vi "Module.Initializer.vi"(4 "StatusTxtBx":refnum<vi>, 5 "Menu Ref":refnum<k9>, 6 "Pane":refnum<vi>, 7 "Main Tab":refnum<vi>, 8 "error in":errorcluster, 9 "Self Ref":refnum<vi>, 10 "Module Config":T3, 11 "SW Rev":T2) -> (0 "error out":errorcluster, 3 "Sys":T1)   [LabVIEW 2024, in "EQMF.lvlib" / "Module Utils.lvlib"]
uses:
  Module Utils.lvlib
  Module Config.ctl
  Queues/Q.Element.ctl
  Module.Working Dirs.ctl
  Module.SW Version Info.ctl
  Module Sys Info.ctl
  Config/Stored Controls/Class.SaveCtrls.lvclass
  Event Log/Event Notification/Event Notification.lvclass
  Config/App Data/Class.AppData.lvclass
  Subscription/Subscription.lvclass
  Queues/Queue Utils.lvlib
  Controls/Controls.lvlib
  Event Log/Event Log.lvlib
  Scheduler/Scheduler.lvlib
  Menu/Menu Utils.lvlib
  Config/Config Utils.lvlib
panel:
  # "Name, PN, Version, Note"
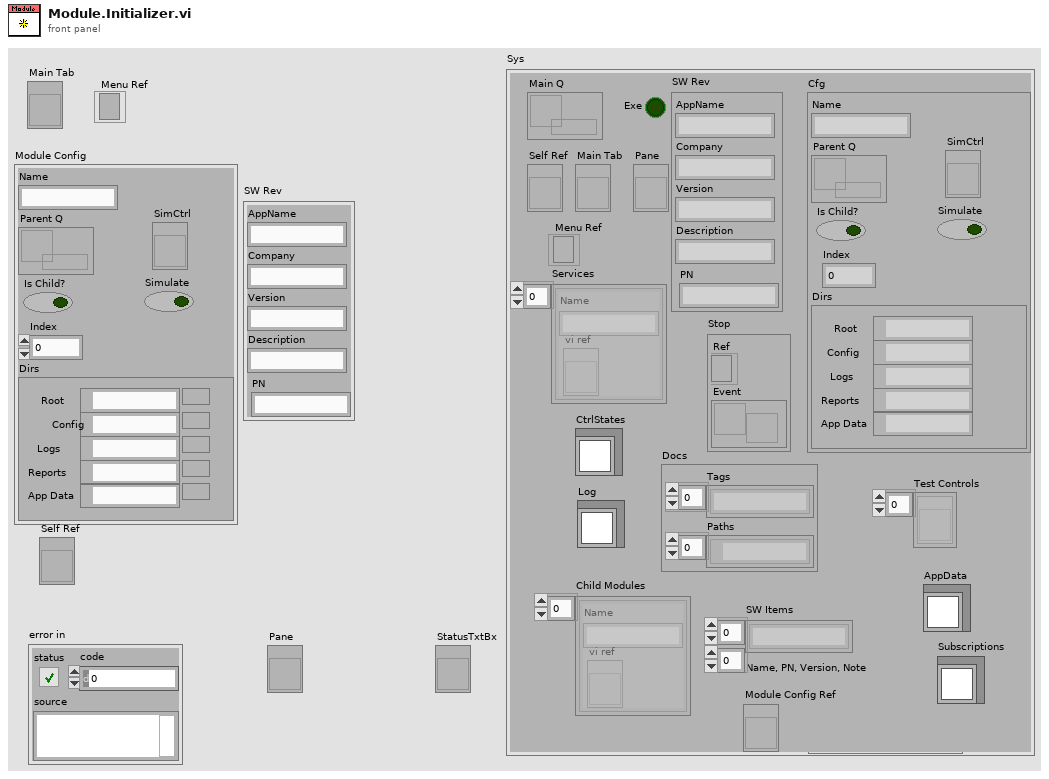
[diagram p1: front panel]
types:
  T1 = typedef "EQMF.lvlib/Module Utils.lvlib/Module Sys Info.ctl" = cluster{"Main Q":refnum<queue>, "Exe":bool, "SW Rev":T2, "Self Ref":refnum<vi>, "Main Tab":refnum<vi>, "Pane":refnum<vi>, "Stop":cluster{"Ref":refnum<event-registration>, "Event":refnum<user-event>}, "Cfg":T3, "Services":cluster{"Name":string, "vi ref":refnum<vi>}[], "Menu Ref":refnum<k9>, "CtrlStates":refnum<class "Class.SaveCtrls.lvclass">, "Docs":cluster{"Tags":string[], "Paths":path[]}, "Log":refnum<class "Event Notification.lvclass">, "Test Controls":refnum<vi>[], "Child Modules":cluster{"Name":string, "vi ref":refnum<vi>}[], "SW Items":string[][], "AppData":refnum<class "Class.AppData.lvclass">, "Subscriptions":refnum<class "Subscription.lvclass">, "Module Config Ref":refnum<vi>}
  T2 = typedef "EQMF.lvlib/Module Utils.lvlib/Module.SW Version Info.ctl" = cluster{"AppName":string, "Company":string, "Version":string, "Description":string, "PN":string}
  T3 = typedef "EQMF.lvlib/Module Utils.lvlib/Module Config.ctl" = cluster{"Name":string, "Parent Q":refnum<queue>, "Is Child?":bool, "Index":i32, "Dirs":T4, "Simulate":bool, "SimCtrl":refnum<vi>}
  T4 = typedef "EQMF.lvlib/Module Utils.lvlib/Module.Working Dirs.ctl" = cluster{"Root":path, "Config":path, "Logs":path, "Reports":path, "App Data":path}
  T5 = enum32{"invalid app kind", "Development System", "Run Time System", "Student Edition", "Embedded LabVIEW", "Evaluation", "Custom"}
  T6 = typedef "LVMenuShortCut.ctl" = cluster{"include Shift key?":bool, "include Ctrl key?":bool, "shortcut key":string}
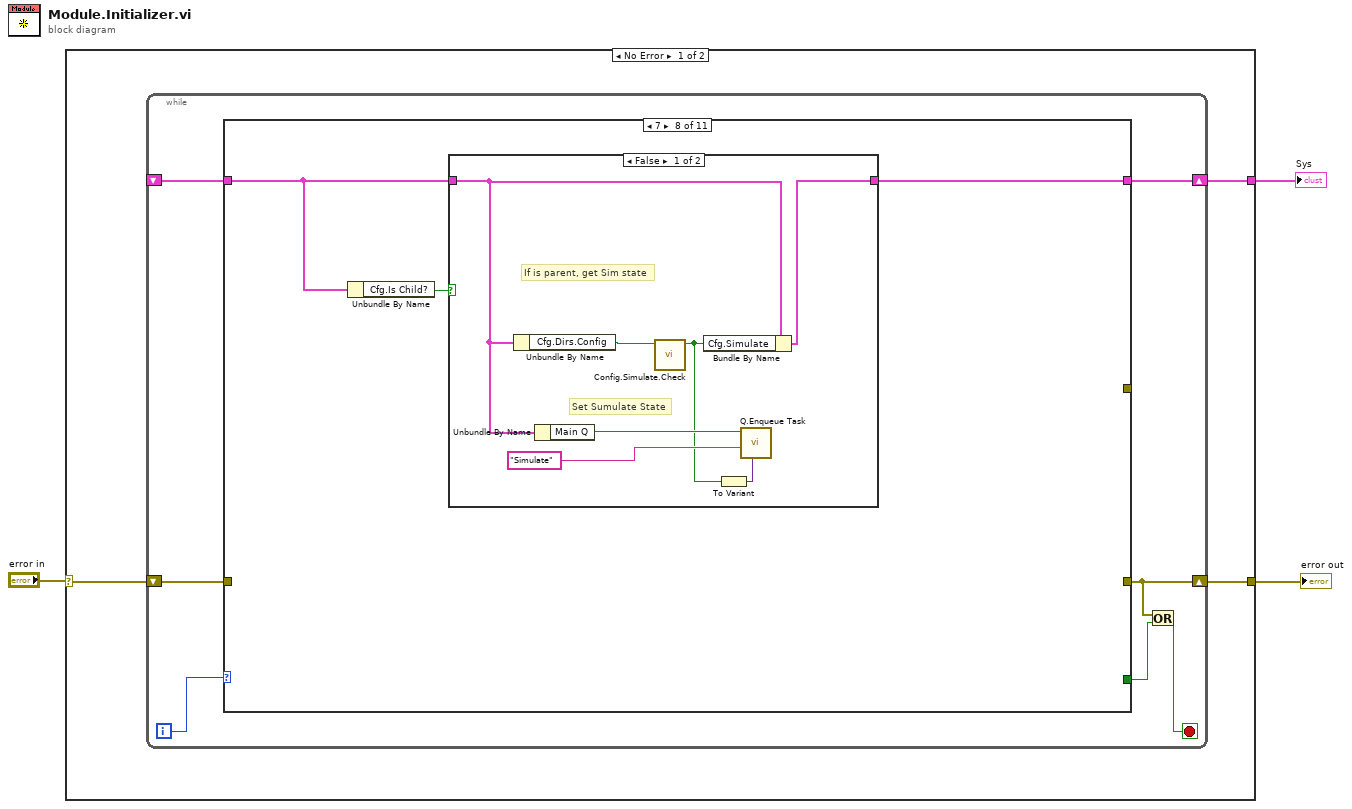
[diagram p0: block diagram]
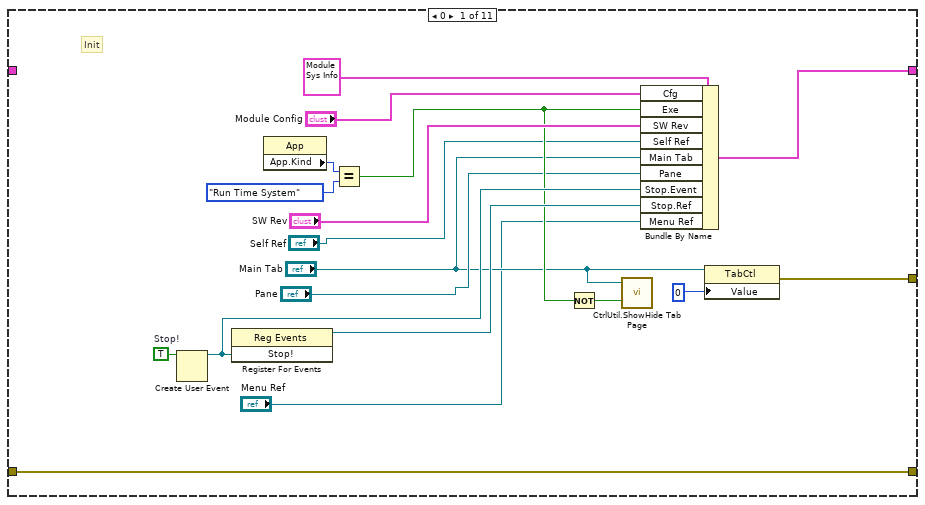
[diagram p2: hidden frame]
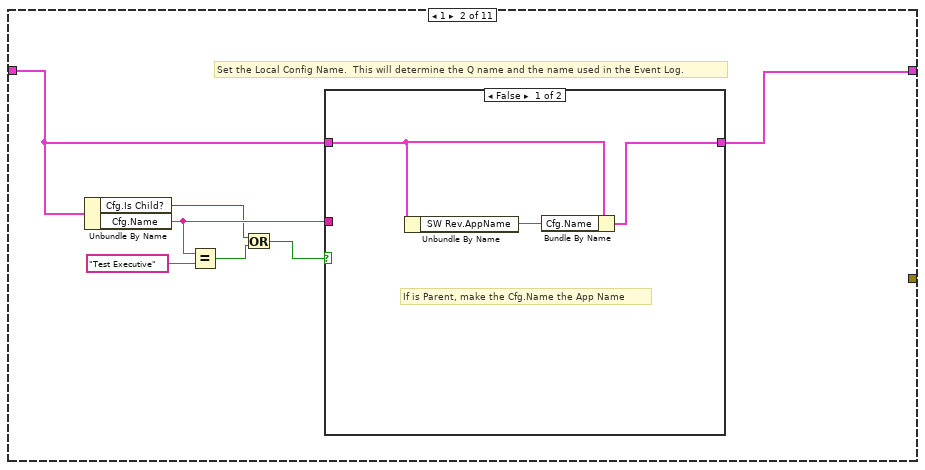
[diagram p3: hidden frame]
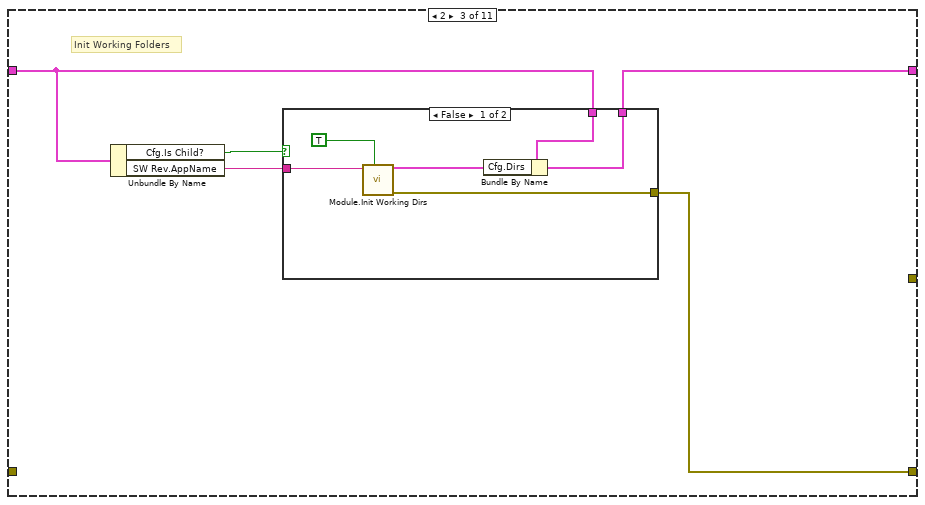
[diagram p5: hidden frame]
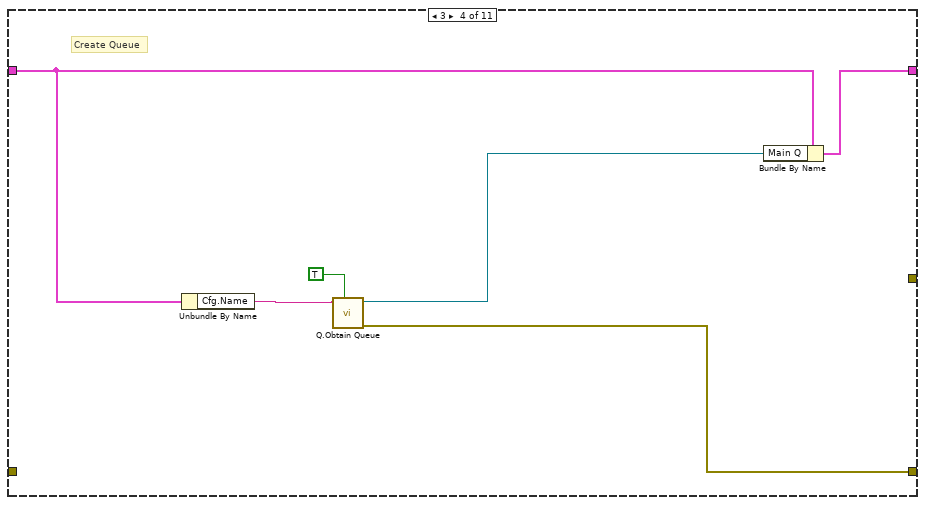
[diagram p7: hidden frame]
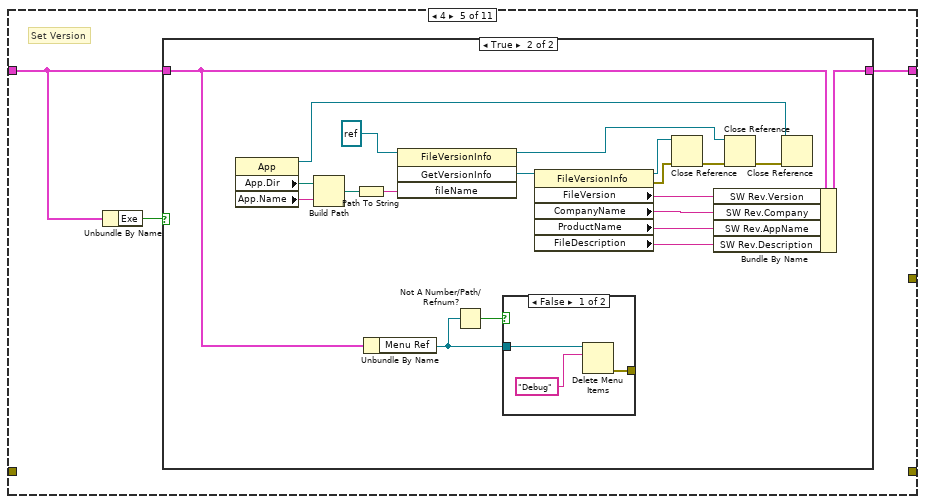
[diagram p8: hidden frame]
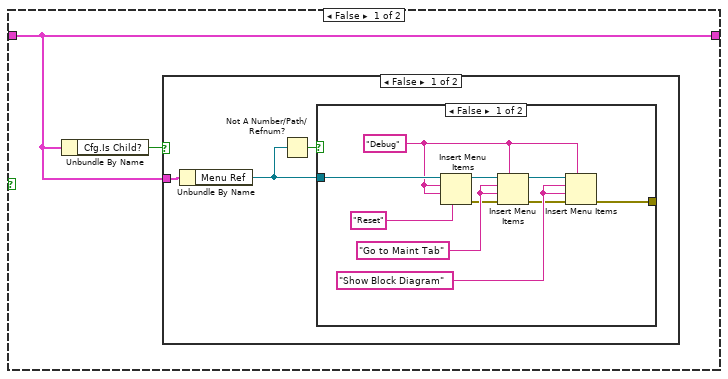
[diagram p9: hidden frame]
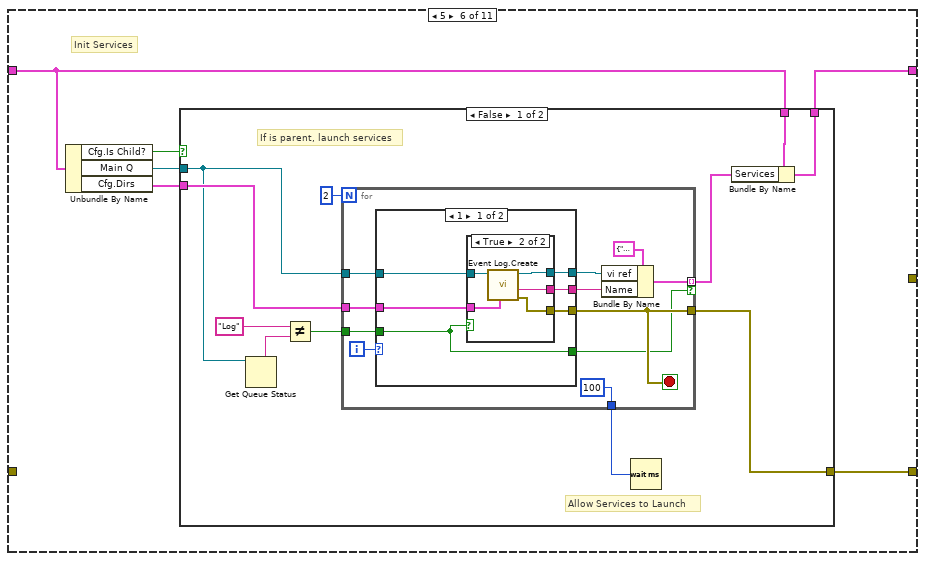
[diagram p13: hidden frame]
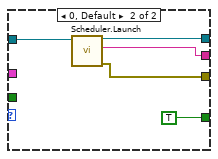
[diagram p15: hidden frame]
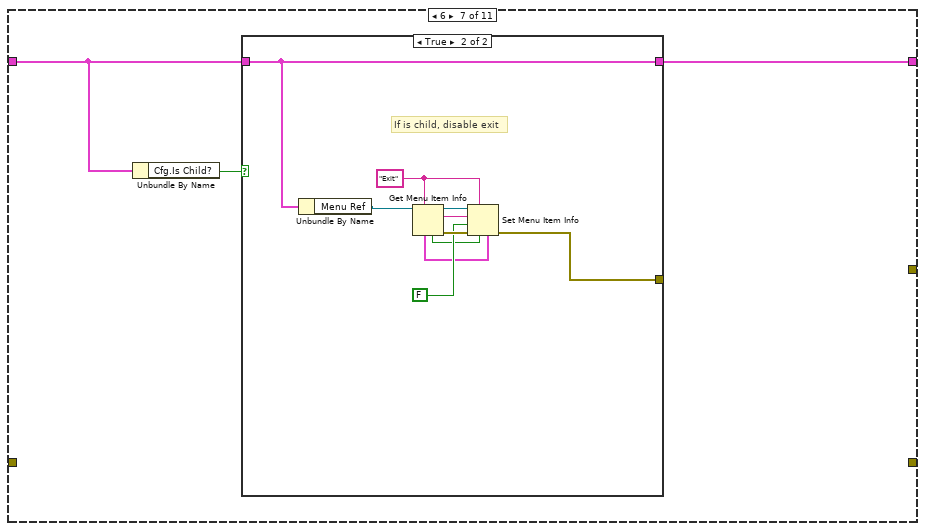
[diagram p17: hidden frame]
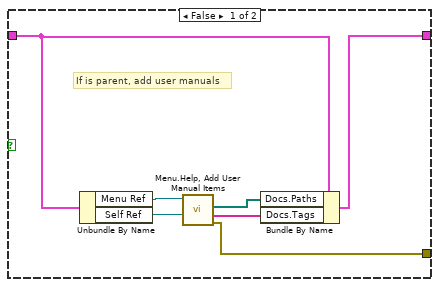
[diagram p18: hidden frame]
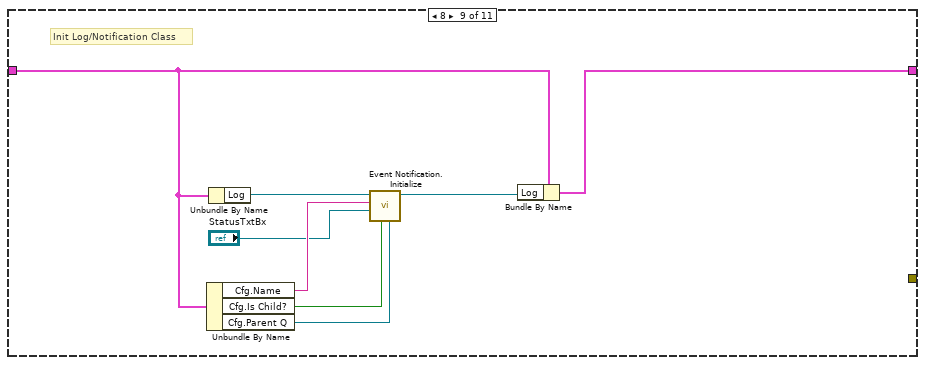
[diagram p20: hidden frame]
diagram:
  n1 = case shown="No Error" "error in" {
    selector: "error in" -> [w6 w197]
    tunnel: [w4 w197] -> w3
    tunnel: [w5 _] -> w1
    frame No Error {
      n2 = while {
        shift-right: [w7] -> w5
        shift-left: _ -> [w12]
        shift-right: [w8] -> w4
        shift-left: w6 -> [w9]
        i -> [w13]
        stop <- w10 stop-if-true
        n3 = case shown="7" w13 {
          tunnel: w12 -> [_ w36 w45 w56 w62 w106 w148 w168 w184 w193 w194]
          tunnel: [_ _ _ _ _ _ _ _ _ _ TRUE] -> w11
          tunnel: w9 -> [w22 _ _ _ _ _ _ _ _ _ w195]
          tunnel: [w22 _ w43 w58 _ w104 _ _ _ _ w195] -> w8
          tunnel: [w26 w35 w44 w60 w61 w105 w149 w169 w185 w192 w194] -> w7
          tunnel: [w15 _ _ _ _ _ _ _ _ _ _] -> _
          frame 0 {
            w25 = TRUE  # Stop!
            # "Init"
            n4 = Create User Event(user event datatype=w25) -> (user event=w24:refnum<user-event>)  [unwired: 1 in, 1 out]
            n5 = register-events(w24) -> (reference out=w23:refnum<event-registration>)  [unwired: 2 in, 1 out]
            n6 = property class="App"() -> ("App.Kind"=w28:T5)  [unwired: 2 in, 2 out]
            n7 = Equal?(x=w28, y=T5."Run Time System" ("Application:Kind")) -> (x = y?=w20:bool)
            n8 = Not(x=w20) -> (.not. x?=w21:bool)
            n9 = call "CtrlUtil.ShowHide Tab Page.vi"("Show"=w21, "Tab Control"="Main Tab") -> ()  [unwired: 3 in]
            n10 = Bundle By Name(cluster=T1 {"Main Q"=refnum, "Exe"=FALSE, "SW Rev"={"AppName"="", "Company"="", "Version"="", "Description"="", "PN"=""}, "Self Ref"=refnum, "Main Tab"=refnum, "Pane"=refnum, "Stop"={"Ref"=refnum, "Event"=refnum}, "Cfg"={"Name"="", "Parent Q"=refnum, "Is Child?"=FALSE, "Index"=0, "Dirs"={"Root"=path "", "Config"=path "", "Logs"=path "", "Reports"=path "", "App Data"=path ""}, "Simulate"=FALSE, "SimCtrl"=refnum}, "Services"=[], "Menu Ref"=refnum, "CtrlStates"=refnum, "Docs"={"Tags"=[], "Paths"=[]}, "Log"=refnum, "Test Controls"=[], "Child Modules"=[], "SW Items"=[], "AppData"=refnum, "Subscriptions"=refnum, "Module Config Ref"=refnum} ("Sys"), "Cfg"="Module Config", "Exe"=w20, "SW Rev"="SW Rev", "Self Ref"="Self Ref", "Main Tab"="Main Tab", "Pane"="Pane", "Stop.Event"=w24, "Stop.Ref"=w23, "Menu Ref"="Menu Ref") -> (w26:T1)
            n11 = property class="TabCtl"(reference="Main Tab", "Value"=0) -> (error out=w15:errorcluster)  [unwired: 1 in, 1 out]
          }
          frame 1 {
            # "Set the Local Config Name.  This will determine the Q name and the name used in the Event Log."
            n12 = Unbundle By Name(w36) -> ("Cfg.Is Child?"=w33:bool, "Cfg.Name"=w37:string)
            n13 = Equal?(x=w37, y="Test Executive") -> (x = y?=w34:bool)
            n14 = Or(x=w33, y=w34) -> (x .or. y?=w32:bool)
            n15 = case shown="False" w32 {
              tunnel: w37 -> [_ _]
              tunnel: w36 -> [w41 w42]
              tunnel: [w39 w42] -> w35
              frame False {
                # "If is Parent, make the Cfg.Name the App Name"
                n16 = Unbundle By Name(w41) -> ("SW Rev.AppName"=w40:string)
                n17 = Bundle By Name(cluster=w41, "Cfg.Name"=w40) -> (w39:T1)
              }
              frame True {
                # "If is Child\n  Use Config name assigned\nIf is Test Executive:\n   No change to Cfg.Name"
              }
            }
          }
          frame 2 {
            # "Init Working Folders"
            n18 = Unbundle By Name(w45) -> ("Cfg.Is Child?"=w46:bool, "SW Rev.AppName"=w47:string)
            n19 = case shown="False" w46 {
              tunnel: w47 -> [w53 _]
              tunnel: [w52 _] -> w43
              tunnel: w45 -> [w50 w54]
              tunnel: [w49 w54] -> w44
              frame False {
                n20 = call "Module.Init Working Dirs.vi"("Public Docs"=TRUE, "App Name"=w53) -> ("error out"=w52:errorcluster, "Working Dirs"=w51:T4)  [unwired: 8 in]
                n21 = Bundle By Name(cluster=w50, "Cfg.Dirs"=w51) -> (w49:T1)
              }
              frame True {
              }
            }
          }
          frame 3 {
            # "Create Queue"
            n22 = Unbundle By Name(w56) -> ("Cfg.Name"=w55:string)
            n23 = call "Q.Obtain Queue.vi"("Enqueue Init"=TRUE, "Q Name"=w55) -> ("error out"=w58:errorcluster, "Q Out"=w59:refnum<queue>)  [unwired: 7 in, 1 out]
            n24 = Bundle By Name(cluster=w56, "Main Q"=w59) -> (w60:T1)
          }
          frame 4 {
            # "Set Version"
            n25 = Unbundle By Name(w62) -> ("Exe"=w63:bool)
            n26 = case shown="True" w63 {
              tunnel: w62 -> [w65 w82]
              tunnel: [w65 w97] -> w61
              frame False {
                n27 = Unbundle By Name(w65) -> ("Cfg.Is Child?"=w64:bool)
                n28 = case shown="False" w64 {
                  tunnel: w65 -> [w68 _]
                  frame False {
                    n29 = Unbundle By Name(w68) -> ("Menu Ref"=w66:refnum<k9>)
                    n30 = Not A Number/Path/Refnum?(number/path/refnum=w66) -> (NaN/Path/Refnum?=w67:bool)
                    n31 = case shown="False" w67 {
                      tunnel: w66 -> [w78 _]
                      tunnel: [w69 _] -> _
                      frame False {
                        w72 = "Show Block Diagram" ("menu tag")
                        w73 = "Go to Maint Tab" ("menu tag")
                        w74 = "Debug" ("menu tag")
                        n32 = Insert Menu Items(4:"Reset" ("after item"), 7:w74, 8:w74, 9:w78) -> (0:w71:errorcluster, 3:w76:refnum<k9>)  [unwired: 2 in, 1 out]
                        n33 = Insert Menu Items(5:w74, 6:w71, 7:w73, 8:w73, 9:w76) -> (0:w70:errorcluster, 3:w75:refnum<k9>)  [unwired: 1 in, 1 out]
                        n34 = Insert Menu Items(5:w74, 6:w70, 7:w72, 8:w72, 9:w75) -> (0:w69:errorcluster)  [unwired: 1 in, 2 out]
                      }
                      frame True {
                      }
                    }
                  }
                  frame True {
                  }
                }
              }
              frame True {
                n35 = property class="App"() -> (reference out=w83:refnum<vi>, "App.Dir"=w88:path, "App.Name"=w87:string)  [unwired: 2 in, 1 out]
                n36 = Build Path(base path=w88, name or relative path=w87) -> (appended path=w86:path)
                n37 = Path To String(path=w86) -> (string=w95:string)
                n38 = Unbundle By Name(w82) -> ("Menu Ref"=w80:refnum<k9>)
                n39 = invoke class="FileVersionInfo" method="GetVersionInfo"(reference=refnum<k24> refnum, "fileName"=w95) -> (reference out=w91:refnum<k24>, "GetVersionInfo"=w98:refnum<k24>)  [unwired: 2 in, 2 out]
                n40 = Not A Number/Path/Refnum?(number/path/refnum=w80) -> (NaN/Path/Refnum?=w79:bool)
                n41 = case shown="False" w79 {
                  tunnel: [w100 _] -> _
                  tunnel: w80 -> [w99 _]
                  frame False {
                    n42 = Delete Menu Items(8:"Debug" ("menu tag"), 9:w99) -> (0:w100:errorcluster)  [unwired: 2 in, 1 out]
                  }
                  frame True {
                  }
                }
                n43 = property class="FileVersionInfo"(reference=w98) -> (reference out=w94:refnum<k24>, error out=w93:errorcluster, "FileVersion"=w96:string, "CompanyName"=w89:string, "ProductName"=w85:string, "FileDescription"=w81:string)  [unwired: 1 in]
                n44 = Close Reference(reference=w94, error in (no error)=w93) -> (error out=w92:errorcluster)
                n45 = Bundle By Name(cluster=w82, "SW Rev.Version"=w96, "SW Rev.Company"=w89, "SW Rev.AppName"=w85, "SW Rev.Description"=w81) -> (w97:T1)
                n46 = Close Reference(reference=w91, error in (no error)=w92) -> (error out=w84:errorcluster)
                n47 = Close Reference(reference=w83, error in (no error)=w84) -> ()  [unwired: 1 out]
              }
            }
          }
          frame 5 {
            # "Init Services"
            n48 = Unbundle By Name(w106) -> ("Cfg.Is Child?"=w107:bool, "Main Q"=w103:refnum<queue>, "Cfg.Dirs"=w102:T4)
            n49 = case shown="False" w107 {
              tunnel: w106 -> [w118 w146]
              tunnel: [w117 w146] -> w105
              tunnel: [w116 _] -> w104
              tunnel: w103 -> [w111 _]
              tunnel: w102 -> [w113 _]
              frame False {
                # "Allow Services to Launch"
                # "If is parent, launch services"
                n50 = Get Queue Status(queue=w111) -> (queue name=w112:string)  [unwired: 2 in, 7 out]
                n51 = Not Equal?(x="Log", y=w112) -> (x != y?=w109:bool)
                n52 = for {
                  N: 2 -> [_]
                  tunnel: [w128] -> w114 mode=indexing if=w122
                  tunnel: [w125] -> w116
                  tunnel: w111 -> [w123]
                  tunnel: w113 -> [w121]
                  tunnel: w109 -> [w120]
                  tunnel: [u32 100 ("milliseconds to wait")] -> w108
                  i -> [w124]
                  stop <- w125 stop-if-true
                  n53 = case shown="1" w124 {
                    tunnel: [w135 w145] -> w129
                    tunnel: [w134 w141] -> w126
                    tunnel: [w133 w144] -> w125
                    tunnel: w123 -> [w132 w143]
                    tunnel: [w130 TRUE] -> w122
                    tunnel: w121 -> [w131 _]
                    tunnel: w120 -> [w130 _]
                    frame 1 {
                      n54 = case shown="True" w130 {
                        tunnel: [_ w140] -> w135
                        tunnel: [_ w139] -> w134
                        tunnel: [_ w138] -> w133
                        tunnel: w132 -> [_ w137]
                        tunnel: w131 -> [_ w136]
                        frame False {
                        }
                        frame True {
                          n55 = call "Event Log.Create.vi"("Working Dirs"=w136, "Q In"=w137) -> ("Error Out"=w138:errorcluster, "Name Out"=w139:string, "reference out"=w140:refnum<vi>)  [unwired: 7 in]
                        }
                      }
                    }
                    frame 0, Default {
                      n56 = call "Scheduler.Launch.vi"("Q In"=w143) -> ("Error Out"=w144:errorcluster, "Name"=w141:string, "VI Refnum"=w145:refnum<vi>)  [unwired: 8 in]
                    }
                  }
                  n57 = Bundle By Name(cluster=cluster{"Name":string, "vi ref":refnum<vi>} {"Name"="", "vi ref"=refnum} ("Service"), "vi ref"=w129, "Name"=w126) -> (w128:cluster{"Name":string, "vi ref":refnum<vi>})
                }
                n58 = Wait (ms)(milliseconds to wait=w108) -> ()  [unwired: 1 out]
                n59 = Bundle By Name(cluster=w118, "Services"=w114) -> (w117:T1)
              }
              frame True {
                # "If is child, then do nothing.  The parent module launched the services"
              }
            }
          }
          frame 6 {
            n60 = Unbundle By Name(w148) -> ("Cfg.Is Child?"=w147:bool)
            n61 = case shown="True" w147 {
              tunnel: w148 -> [w155 w163]
              tunnel: [w154 w163] -> w149
              tunnel: [w150 w157] -> _
              frame False {
                # "If is parent, add user manuals"
                n62 = Unbundle By Name(w155) -> ("Menu Ref"=w151:refnum<k9>, "Self Ref"=w156:refnum<vi>)
                n63 = call "Menu.Help, Add User Manual Items.vi"("Main VI"=w156, "Menu Ref"=w151) -> ("error out"=w150:errorcluster, "Tags"=w152:string[], "Paths"=w153:path[])  [unwired: 6 in, 1 out]
                n64 = Bundle By Name(cluster=w155, "Docs.Paths"=w153, "Docs.Tags"=w152) -> (w154:T1)
              }
              frame True {
                w161 = "Exit" ("item tag")
                # "If is child, disable exit"
                n65 = Unbundle By Name(w163) -> ("Menu Ref"=w162:refnum<k9>)
                n66 = Get Menu Item Info(7:w161, 11:w162) -> (0:w165:errorcluster, 2:w160:string, 3:w166:refnum<k9>, 4:w158:bool, 6:w159:T6)  [unwired: 1 in, 2 out]
                n67 = Set Menu Item Info(4:w159, 6:w158, 7:w161, 8:w165, 9:FALSE, 10:w160, 11:w166) -> (0:w157:errorcluster)  [unwired: 1 out]
              }
            }
          }
          frame 7 {
            n68 = Unbundle By Name(w168) -> ("Cfg.Is Child?"=w167:bool)
            n69 = case shown="False" w167 {
              tunnel: w168 -> [w174 w177]
              tunnel: [w176 w177] -> w169
              frame False {
                # "Set Sumulate State"
                # "If is parent, get Sim state"
                n70 = Unbundle By Name(w174) -> ("Cfg.Dirs.Config"=w175:path)
                n71 = Unbundle By Name(w174) -> ("Main Q"=w173:refnum<queue>)
                n72 = call "Config.Simulate.Check.vi"("Config Folder"=w175) -> ("Simulate"=w170:bool)  [unwired: 10 in]
                n73 = Bundle By Name(cluster=w174, "Cfg.Simulate"=w170) -> (w176:T1)
                n74 = To Variant(anything=w170) -> (Variant=w171:variant)
                n75 = call "Q.Enqueue Task.vi"("Data1"=w171, "Task Name"="Simulate", "Q In"=w173) -> ()  [unwired: 7 in, 2 out]
              }
              frame True {
                # "Do nothing if is child"
              }
            }
          }
          frame 8 {
            # "Init Log/Notification Class"
            n76 = Unbundle By Name(w184) -> ("Cfg.Name"=w181:string, "Cfg.Is Child?"=w179:bool, "Cfg.Parent Q"=w178:refnum<queue>)
            n77 = Unbundle By Name(w184) -> ("Log"=w183:refnum<class "Event Notification.lvclass">)
            n78 = call "Event Notification.Initialize.vi"("Parent Q"=w178, "Is Child?"=w179, "StatusTxtBoxRef"="StatusTxtBx", "AppID"=w181, "Event Notification in"=w183) -> ("Event Notification out"=w182:refnum<class "Event Notification.lvclass">)  [unwired: 5 in, 1 out]
            n79 = Bundle By Name(cluster=w184, "Log"=w182) -> (w185:T1)
          }
          frame 9 {
            w188 = ""  # PN
            # "PN will need to be specified by modifying this item in the application's code."
            # "Name, PN, Ver, Note"
            n80 = Unbundle By Name(w193) -> ("SW Rev.AppName"=w189:string, "SW Rev.Version"=w187:string, "SW Rev.Description"=w186:string)  [unwired: 1 out]
            n81 = Build Array(w189, w188, w187, w186) -> (w191:string[])
            n82 = Build Array(w191) -> (w190:string[][])
            n83 = Bundle By Name(cluster=w193, "SW Items"=w190) -> (w192:T1)
          }
          frame Default {
            # "Done"
          }
        }
        n84 = Or(x=w8, y=w11) -> (x .or. y?=w10:bool)
      }
    }
    frame Error {
    }
  }
  "error out" <- w3
  "Sys" <- w1
